vi "ZL300 Wait for Move.vi"(0 "Axis In":u32, 2 "Threshold":dbl=0.002 format="%#_13g", 5 "Handle In":i32, 11 "Error In":errorcluster) -> (4 "Axis Out":u32, 6 "Handle Out":i32, 8 "Position":dbl, 15 "Error Out":errorcluster)   [LabVIEW 2020]
uses:
  MCL Libraries/Madlib.dll
panel:
  out "Pos":dbl[](graph)
  out "Diff":dbl[](graph)
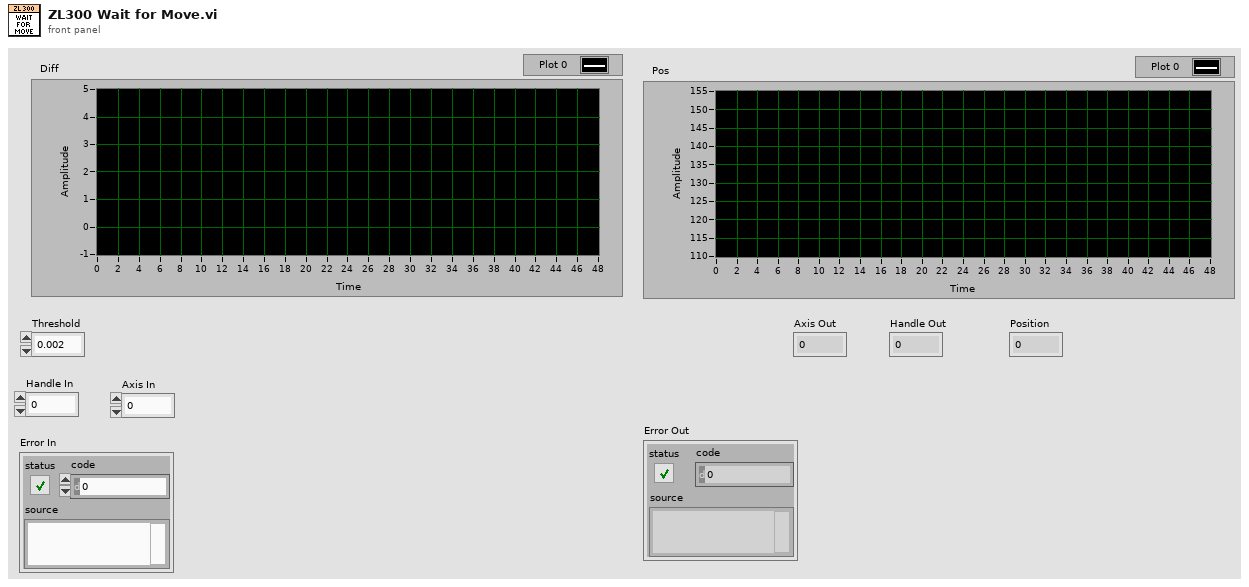
[diagram p1: front panel]
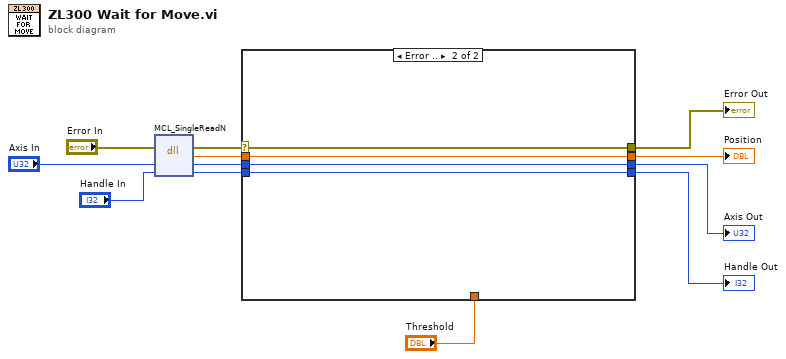
[diagram p0: block diagram]
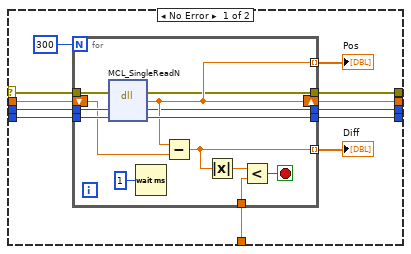
[diagram p2: hidden frame]
diagram:
  n1 = dll-call lib="C:/Users/George Sirinakis/Documents/Microscope-Control/Device Library/Stages/Mad City Labs/ZL300/MCL Libraries/MADLib.dll" fn="MCL_SingleReadN" label="SingleReadN"(error in="Error In", "Axis"="Axis In", "Handle"="Handle In") -> (error out=w6:errorcluster, "Position"=w5:dbl, "Axis"=w4:u32, "Handle"=w3:i32)  [unwired: 2 in, 1 out]
  n2 = case shown="Error .." w6 {
    selector: w6 -> [w16 w41]
    tunnel: [w21 w38] -> w12
    tunnel: w3 -> [w13 w39]
    tunnel: w4 -> [w14 w40]
    tunnel: [w20 w40] -> w10
    tunnel: [w19 w39] -> w9
    tunnel: [w18 w41] -> w11
    tunnel: "Threshold" -> [w17 _]
    tunnel: w5 -> [w15 w38]
    frame No Error {
      n3 = for {
        N: 300 -> [_]
        shift-right: [w29] -> w21
        shift-left: w15 -> [w35]
        tunnel: w14 -> [w37]
        tunnel: w13 -> [w36]
        tunnel: [w31] -> w23 mode=indexing
        tunnel: [w30] -> w19
        tunnel: [w29] -> w22 mode=indexing
        tunnel: [w28] -> w20
        tunnel: w16 -> [w27]
        tunnel: [w26] -> w18
        tunnel: w17 -> [w25]
        stop <- w32 stop-if-true
        n4 = dll-call lib="C:/Users/George Sirinakis/Documents/Microscope-Control/Device Library/Stages/Mad City Labs/ZL300/MCL Libraries/MADLib.dll" fn="MCL_SingleReadN" label="SingleReadN"(error in=w27, "Axis"=w37, "Handle"=w36) -> (error out=w26:errorcluster, "Position"=w29:dbl, "Axis"=w28:u32, "Handle"=w30:i32)  [unwired: 2 in, 1 out]
        n5 = Wait (ms)(milliseconds to wait=u32 1) -> ()  [unwired: 1 out]
        n6 = Subtract(x=w29, y=w35) -> (x-y=w31:dbl)
        n7 = Absolute Value(x=w31) -> (abs(x)=w33:dbl)
        n8 = Less?(x=w33, y=w25) -> (x < y?=w32:bool)
      }
      "Diff" <- w23
      "Pos" <- w22
    }
    frame Error {
    }
  }
  "Position" <- w12
  "Error Out" <- w11
  "Handle Out" <- w9
  "Axis Out" <- w10
